vi "hidSPD Read SPD Name.vi"(8 "error in (no error)":errorcluster, 11 "spdDevSession in":T1 {"hidSPD.Sturtup Values"."HV_bias" format="%#_6p, V"; "hidSPD.Sturtup Values"."TSet" format="%#_6p, DegC"; "hidSPD.Controller"."HV_bias" format="%#_6p, V"; "hidSPD.Controller"."TSet" format="%#_6p, DegC"}) -> (0 "error out":errorcluster, 2 "Name":string, 3 "spdDevSession out":T1 {"hidSPD.Sturtup Values"."HV_bias" format="%#_6p, V"; "hidSPD.Sturtup Values"."TSet" format="%#_6p, DegC"; "hidSPD.Controller"."HV_bias" format="%#_6p, V"; "hidSPD.Controller"."TSet" format="%#_6p, DegC"})   [LabVIEW 2018, in "hidSPDLibForLabView.lvlib"]
uses:
  hidSPDLibForLabView.lvlib
  hidSPD Controls/hidSPD Device Session.ctl
  hidSPD Controls/hidSPD Controller.ctl
  hidSPD Controls/hidSPD SPD Type.ctl
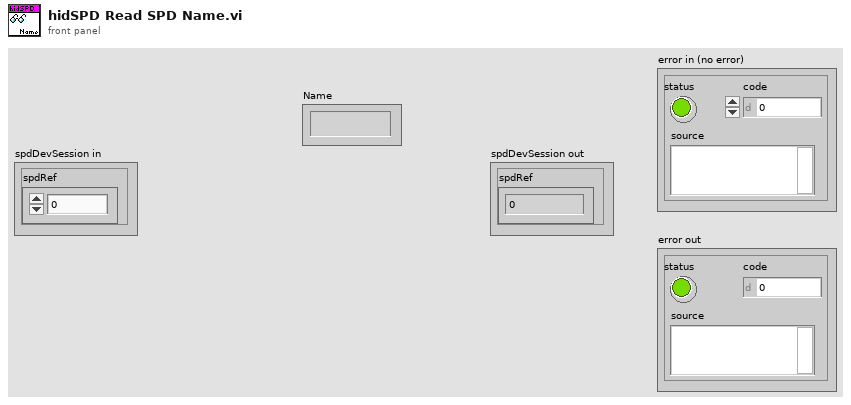
[diagram p1: front panel]
types:
  T1 = typedef "hidSPDLibForLabView.lvlib/hidSPD Device Session.ctl" = cluster{"spdRef":u64, "connected":bool, "spdName":string, "hidSPD.Controller":T2, "hidSPD.Sturtup Values":T2, "SPD Type":T3}
  T2 = typedef "hidSPDLibForLabView.lvlib/hidSPD Controller.ctl" = cluster{"TSet":sgl, "HV_bias":sgl, "DDS_stb_code":u16}
  T3 = typedef "hidSPDLibForLabView.lvlib/hidSPD SPD Type.ctl" = enum16{"Free Run", "Gate"}
  T4 = enum16{"big-endian, network order", "native, host order", "little-endian"}
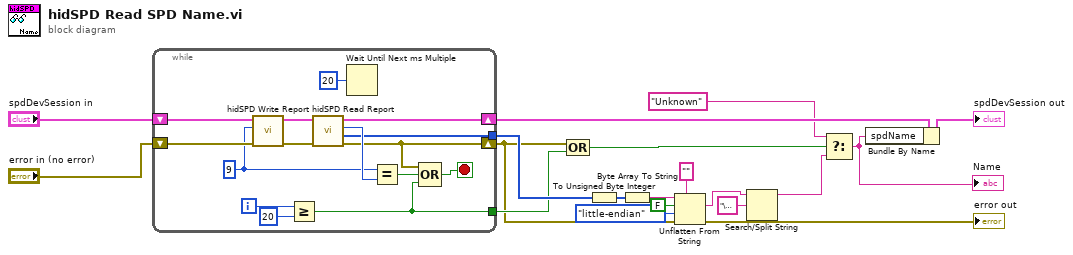
[diagram p0: block diagram]
diagram:
  n1 = while {
    shift-right: [w34] -> w18
    shift-left: "spdDevSession in" -> [w27]
    tunnel: [w31] -> w16
    shift-right: [w29] -> w4
    shift-left: "error in (no error)" -> [w26]
    tunnel: [w20] -> w8
    i -> [w22]
    stop <- w28 stop-if-true
    w25 = 9 ("cmd")
    n2 = call "hidSPD Write Report.vi"("error in (no error)"=w26, "cmd"=w25, "spdDevSession in"=w27) -> ("error out"=w24:errorcluster, "spdDevSession out"=w23:T1)  [unwired: 7 in]
    n3 = Greater Or Equal?(x=w22, y=20) -> (x >= y?=w20:bool)
    n4 = call "hidSPD Read Report.vi"("error in (no error)"=w24, "spdDevSession in"=w23) -> ("error out"=w29:errorcluster, "data"=w31:i32[], "cmd"=w32:i32, "spdDevSession out"=w34:T1)  [unwired: 6 in]
    n5 = Wait Until Next ms Multiple(millisecond multiple=u32 20) -> ()  [unwired: 1 out]
    n6 = Equal?(x=w25, y=w32) -> (x = y?=w30:bool)
    n7 = Compound Arithmetic op=OR(w29, w30, w20) -> (w28:bool)
  }
  n8 = Compound Arithmetic op=OR(w4, w8) -> (w5:bool)
  n9 = To Unsigned Byte Integer(number=w16) -> (unsigned 8bit integer=w15:u8[])
  n10 = Byte Array To String(unsigned byte array=w15) -> (string=w14:string)
  n11 = Unflatten From String(type="", binary string=w14, data includes array or string size? (T)=FALSE, byte order (0:big-endian, network order)=T4."little-endian", error in (no error)=w4) -> (value=w2:string, error out=→"error out":errorcluster)  [unwired: 1 out]
  n12 = Search/Split String(string=w2, search string/char (-)="\u0000") -> (substring before match=w1:string)  [unwired: 1 in, 2 out]
  n13 = Select(t="Unknown", s=w5, f=w1) -> (s? t:f=w6:string)
  "Name" <- w6
  n14 = Bundle By Name(cluster=w18, "spdName"=w6) -> (→"spdDevSession out":T1)
